vi "http parse header.vi"(9 "transmit queue":refnum<queue>, 10 "data in":string, 11 "application request":T1) -> (2 "abort":bool, 3 "application request out":T1)   [LabVIEW 2013]
uses:
  http request.ctl
  http method.ctl
  http response.ctl
  http response packet type.ctl
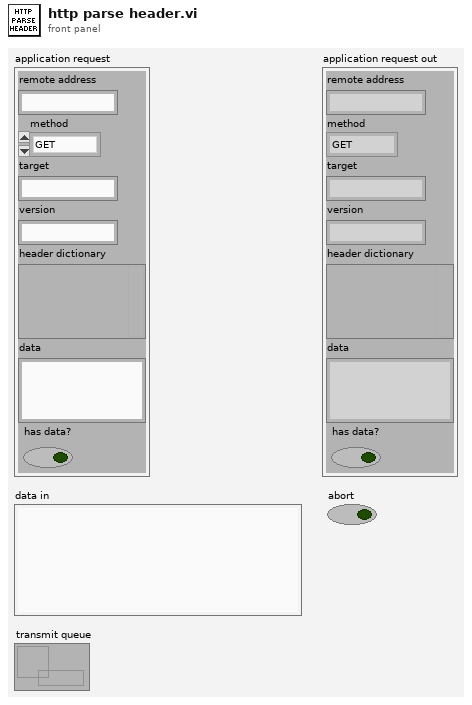
[diagram p1: front panel]
types:
  T1 = typedef "http request.ctl" = cluster{"remote address":string, "method":T2, "target":string, "version":string, "header dictionary":variant, "data":string, "has data?":bool}
  T2 = typedef "http method.ctl" = enum16{"GET", "POST", "PUT", "DELETE", "HEAD", "OPTIONS", "upgrade"}
  T3 = typedef "http response.ctl" = cluster{"packet type":T4, "version":string, "reason code":u16, "status string":string, "header dictionary":variant, "cookies":string[], "data":string}
  T4 = typedef "http response packet type.ctl" = enum16{"full response", "header only", "data only", "last data"}
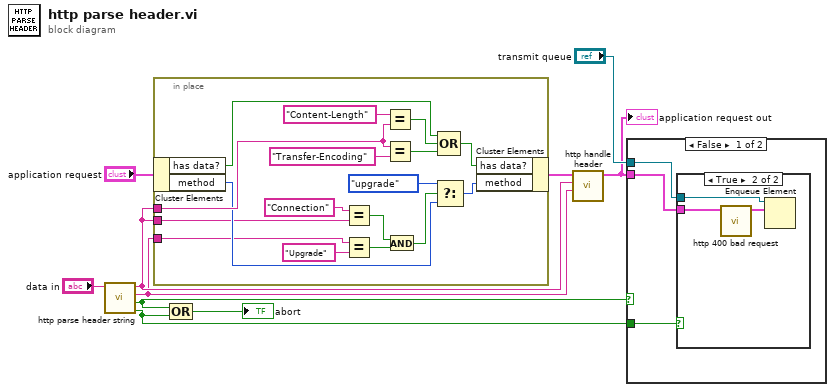
[diagram p0: block diagram]
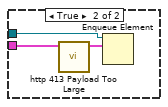
[diagram p3: hidden frame]
diagram:
  n1 = call "http parse header string.vi"("raw string"="data in") -> ("no field name"=w6:bool, "no crlf"=w5:bool, "header field data"=w1:string, "header field name"=w2:string)  [unwired: 7 in]
  n2 = in-place {
    in-place-border: w2 -> [w21]
    in-place-border: w2 -> [w12]
    in-place-border: w1 -> [w11]
    n3 = in-place-cluster #1("application request") -> ("has data?"=w23:bool, "method"=w15:T2)
    n4 = Equal?(x="Connection" ("name"), y=w12) -> (x = y?=w17:bool)
    n5 = Equal?(x=w11, y="Upgrade" ("name")) -> (x = y?=w18:bool)
    n6 = Equal?(x="Content-Length" ("name"), y=w21) -> (x = y?=w26:bool)
    n7 = Equal?(x=w21, y="Transfer-Encoding" ("name")) -> (x = y?=w27:bool)
    n8 = And(x=w17, y=w18) -> (x .and. y?=w16:bool)
    n9 = Select(t=http_method."upgrade", s=w16, f=w15) -> (s? t:f=w14:T2)
    n10 = Compound Arithmetic op=OR(w23, w26, w27) -> (w22:bool)
    n11 = in-place-cluster #1("has data?"=w22, "method"=w14) -> (w4:T1)
  }
  n12 = Compound Arithmetic op=OR(w5, w6) -> (→"abort":bool)
  n13 = call "http handle header.vi"("header field data"=w1, "header field name"=w2, "application request in"=w4) -> ("application request out"=w3:T1)  [unwired: 8 in]
  "application request out" <- w3
  n14 = case shown="False" w5 {
    tunnel: "transmit queue" -> [w30 w36]
    tunnel: w6 -> [w29 _]
    tunnel: w3 -> [w28 w34]
    frame False {
      n15 = case shown="True" w29 {
        tunnel: w30 -> [_ w33]
        tunnel: w28 -> [_ w32]
        frame False {
        }
        frame True {
          n16 = call "http 400 bad request.vi"("application request in"=w32) -> ("application request out"=w31:T3)  [unwired: 10 in]
          n17 = Enqueue Element(queue=w33, element=w31) -> ()  [unwired: 2 in, 3 out]
        }
      }
    }
    frame True {
      n18 = call "http 413 Payload Too Large.vi"("application request in"=w34) -> ("application request out"=w35:T3)  [unwired: 10 in]
      n19 = Enqueue Element(queue=w36, element=w35) -> ()  [unwired: 2 in, 3 out]
    }
  }
